vi "Test Control Gripper Logic.vi"() -> ()   [LabVIEW 2014]
panel:
  in  "Open Gripper":bool
  out "State of Close Gripper":bool
  in  "Close Gripper":bool
  in  "stop":bool
  out "State of Open Gripper":bool
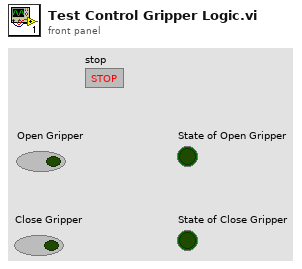
[diagram p1: front panel]
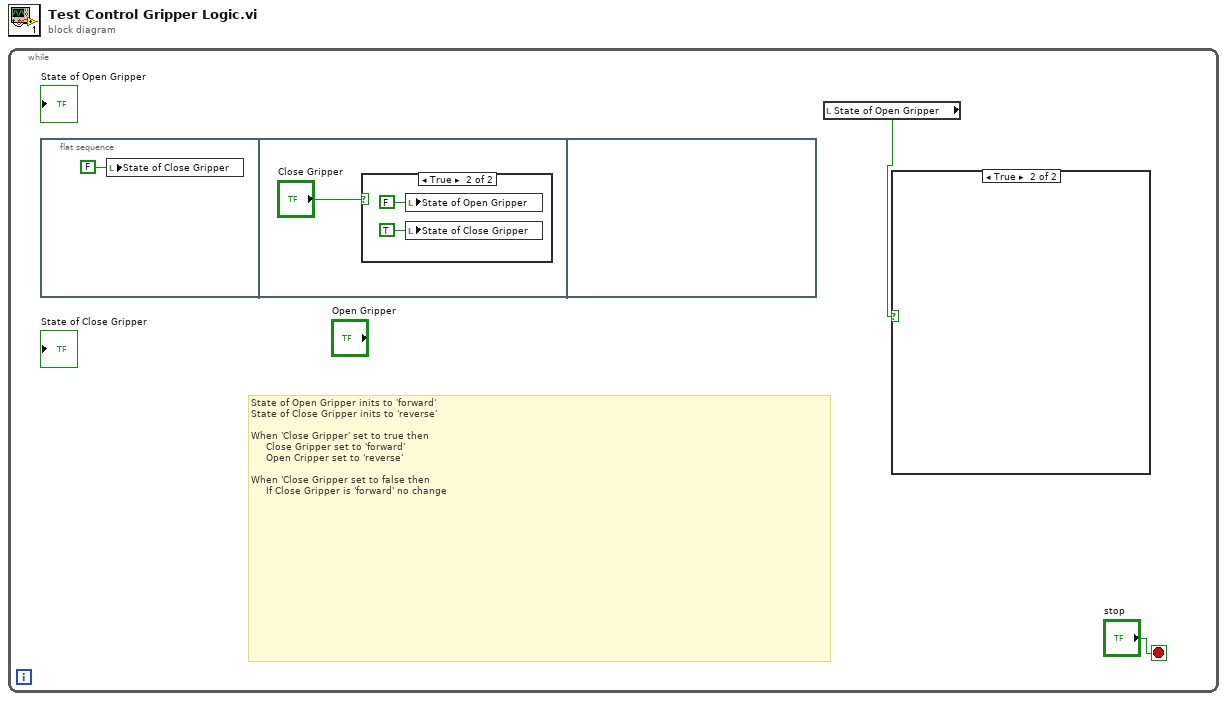
[diagram p0: block diagram]
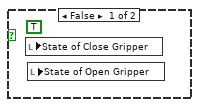
[diagram p3: hidden frame]
diagram:
  n1 = while {
    stop <- "stop" stop-if-true
    # "State of Open Gripper inits to 'forward'\nState of Close Gripper inits to 'reverse'\n\nWhen 'Close Gripper' set to true then \n     Close Gripper set to 'forward'\n     Open Cripper set to 'reverse'\n\nWhen 'Close Gripper set to false then\n     If Close Gripper is 'forward' no change"
    n2 = flat-sequence {
      frame #0 {
        n3 = local write "State of Close Gripper"(FALSE) -> ()
      }
      frame #1 {
        n4 = case shown="True" "Close Gripper" {
          frame False {
            (unwired) TRUE
            n5 = local read "State of Close Gripper"() -> ()  [unwired: 1 in]
            n6 = local read "State of Open Gripper"() -> ()  [unwired: 1 in]
          }
          frame True {
            n7 = local write "State of Open Gripper"(FALSE) -> ()
            n8 = local write "State of Close Gripper"(TRUE) -> ()
          }
        }
      }
      frame #2 {
      }
    }
    n9 = local read "State of Open Gripper"() -> (w1:bool)
    n10 = case shown="True" w1 {
      frame False {
      }
      frame True {
      }
    }
  }
